vi "_Parse IEM List Margin Result.vi"(8 "error in (no error)":errorcluster, 10 "Input String":string, 11 "VISA resource name":refnum<visa-resource-name>) -> (0 "error out":errorcluster, 1 "Results":T1(array[cluster]) {"Margin" format="%^.3e"; "Carrier Leakage" format="%^.3e"; "IQ Image" format="%^.3e"}, 2 "Reliability":i32, 3 "VISA resource name out":refnum<visa-resource-name>)   [LabVIEW 2020, in "Rohde&Schwarz CMWXP NR FR1 Measurement.lvlib"]
uses:
  <instrlib>/Rohde&Schwarz CMWXP NR FR1 Measurement/Rohde&Schwarz CMWXP NR FR1 Measurement.lvlib
  <instrlib>/Rohde&Schwarz CMWXP NR FR1 Measurement/Private/rsidr_core.llb/rsidr_core.lvlib
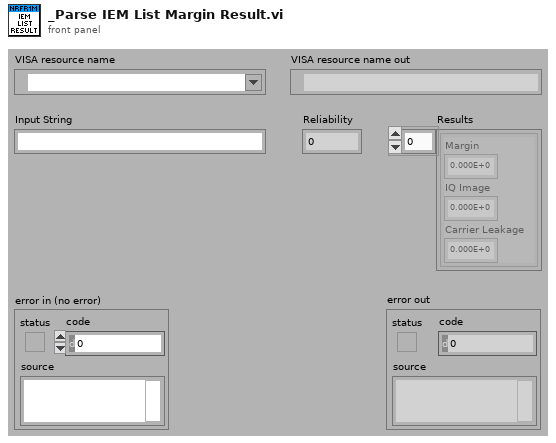
[diagram p1: front panel]
types:
  T1 = cluster{"Margin":dbl, "IQ Image":dbl, "Carrier Leakage":dbl}[]
  T2 = cluster{"Margin":dbl, "IQ Image":dbl, "Carrier Leakage":dbl}
  T3 = cluster{"double array out[0]":dbl, "double array out[1]":dbl, "double array out[2]":dbl}
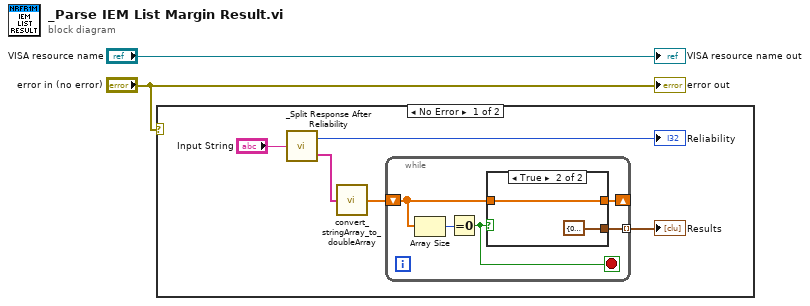
[diagram p0: block diagram]
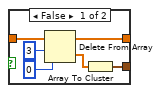
[diagram p2: hidden frame]
diagram:
  n1 = case shown="No Error" "error in (no error)" {
    frame No Error {
      n2 = call <instrlib>:"_Split Response After Reliability.vi"("Input String"="Input String") -> ("Response out"=w5:string[], "Reliability out"=→"Reliability":i32)
      n3 = call <instrlib>:"convert_stringArray_to_doubleArray.vi"("string array in"=w5) -> ("double array out"=w4:dbl[])  [unwired: 4 in]
      n4 = while {
        shift-right: [w9] -> _
        shift-left: w4 -> [w10]
        tunnel: [w8] -> w3 mode=indexing
        stop <- w11 stop-if-true
        n5 = Array Size(array=w10) -> (size(s)=w12:i32)
        n6 = Equal To 0?(x=w12) -> (x = 0?=w11:bool)
        n7 = case shown="True" w11 {
          tunnel: w10 -> [w18 w20]
          tunnel: [w14 w20] -> w9
          tunnel: [w13 T2 {"Margin"=0.0, "IQ Image"=0.0, "Carrier Leakage"=0.0} ("Result")] -> w8
          frame False {
            n8 = Delete From Array(array=w18, length=3, index=0) -> (deleted portion=w15:dbl[], array with subset deleted=w14:dbl[])
            n9 = Array To Cluster(array=w15) -> (cluster=w13:T3)
          }
          frame True {
          }
        }
      }
      "Results" <- w3
    }
    frame Error {
    }
  }
  "VISA resource name out" <- "VISA resource name"
  "error out" <- "error in (no error)"
